vi "Get Configured Backend.vi"(8 "error in (no error)":errorcluster) -> (0 "error out":errorcluster, 3 "Backend":T1=enum."Null")   [LabVIEW 2020, in "G-Audio.lvlib"]
doc: "Get the currently configured backend.\n\nBackend will be Null if the backend hasn't been configured (with Configure Audio Device.vi) or has been cleared (with Clear Audio Backend.vi)."
uses:
  G-Audio.lvlib
  Controls/Backends.ctl
  <vilib>/Utility/error.llb/Error Cluster From Error Code.vi
  lib/g_audio_32.dll
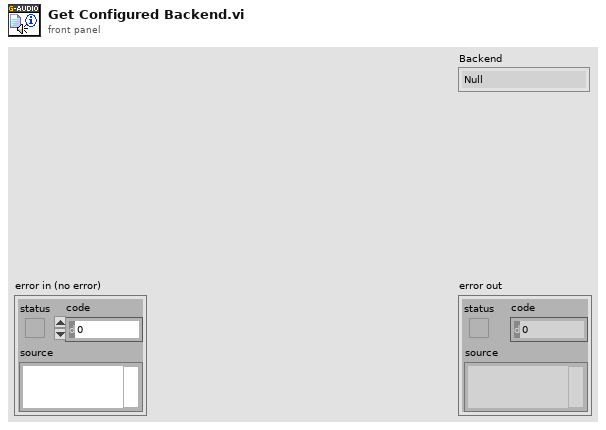
[diagram p1: front panel]
types:
  T1 = typedef "G-Audio.lvlib/Backends.ctl" = enum16{"WASAPI", "DirectSound", "WinMM", "Core Audio", "sndio", "audio(4)", "OSS", "PulseAudio", "ALSA", "JACK", "AAudio", "OpenSL|ES", "Web Audio", "Custom", "Null", "Default"}
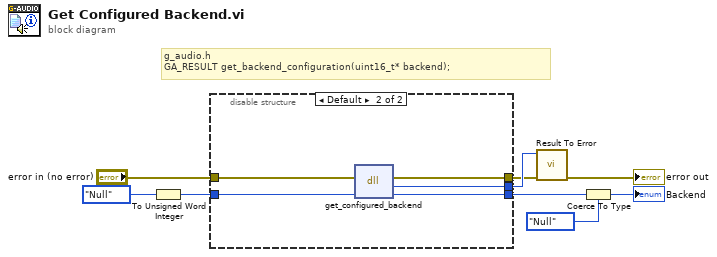
[diagram p0: block diagram]
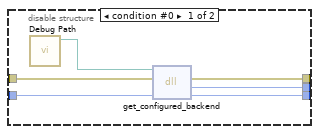
[diagram p2: hidden frame]
diagram:
  # "g_audio.h\nGA_RESULT get_backend_configuration(uint16_t* backend);"
  n1 = To Unsigned Word Integer(number=Backends."Null" ("Backends")) -> (unsigned 16bit integer=w4:u16)
  n2 = disable-structure shown="Default" {
    disable-tunnel: "error in (no error)" -> [w15 w20]
    disable-tunnel: w4 -> [w11 w19]
    disable-tunnel: [w14 w18] -> w8
    disable-tunnel: [w13 w17] -> w9
    disable-tunnel: [w10 w16] -> w3
    frame condition #0 {
      n3 = call "Debug Path.vi"() -> ("Debug Path"=w12:path)  [unwired: 11 in]
      n4 = dll-call lib="?" fn="get_configured_backend"(path in=w12, error in=w15, "backend"=w11) -> (error out=w14:errorcluster, "result"=w13:i32, "backend"=w10:u16)  [unwired: 1 in, 1 out]
    }
    frame condition #1 (active) {
      n5 = dll-call lib="C:/github/dataflowg/g-audio/src/LabVIEW/G-Audio/lib/g_audio_*.*" fn="get_configured_backend"(error in=w20, "backend"=w19) -> (error out=w18:errorcluster, "result"=w17:i32, "backend"=w16:u16)  [unwired: 2 in, 1 out]
    }
  }
  n6 = call "Result To Error.vi"("error in (no error)"=w8, "Result Code"=w9) -> ("error out"=→"error out":errorcluster)  [unwired: 9 in]
  n7 = Coerce To Type(0:w3, 1:Backends."Null" ("Backends")) -> (2:→"Backend":T1)
